vi "DC_CNTRL_step_HV.vi"(0 "Handle":u64, 1 "Ignore NACK":bool, 2 "Read Answer?":bool, 3 "Clear  RxTx Buffer?":bool, 5 "Box Number":u16(ring), 7 "Step (V)":dbl, 9 "Max Range (V)":dbl, 11 "error in (no error)":errorcluster) -> (4 "Handle out":u64, 15 "error out":errorcluster)   [LabVIEW 2019]
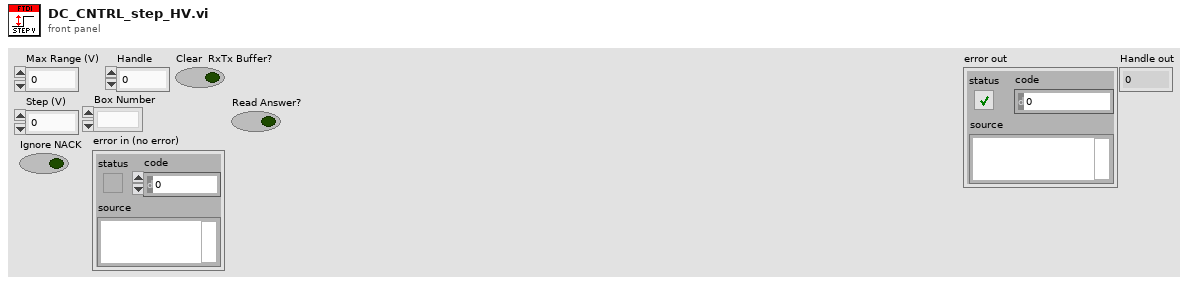
[diagram p1: front panel]
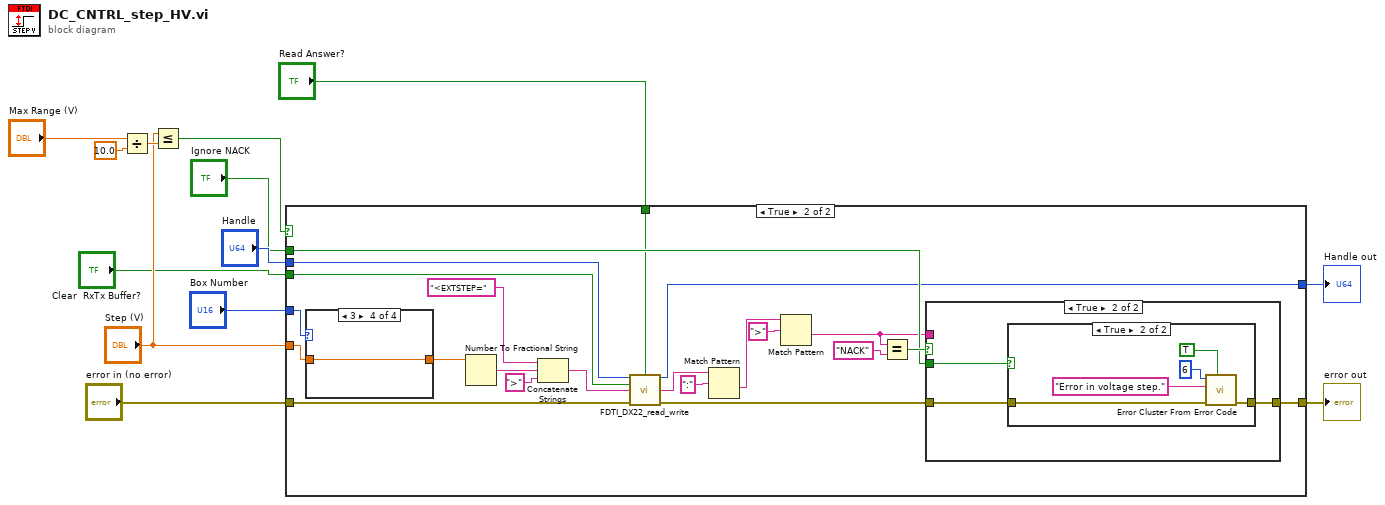
[diagram p0: block diagram]
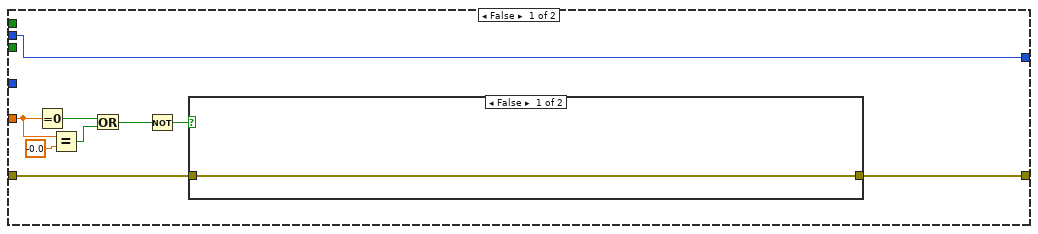
[diagram p2: hidden frame]
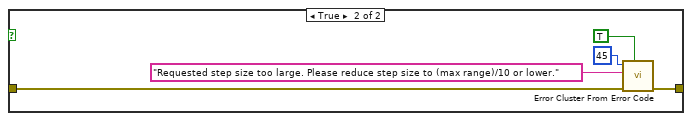
[diagram p3: hidden frame]
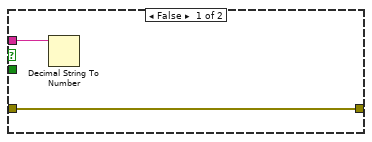
[diagram p4: hidden frame]
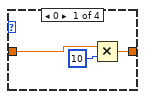
[diagram p6: hidden frame]
diagram:
  n1 = Divide(x="Max Range (V)", y=10.0) -> (x/y=w11:dbl)
  n2 = Less Or Equal?(x="Step (V)", y=w11) -> (x <= y?=w10:bool)
  n3 = case shown="True" w10 {
    tunnel: "Handle" -> [w14 w44]
    tunnel: "Box Number" -> [_ w50]
    tunnel: "Step (V)" -> [w21 w49]
    tunnel: "Ignore NACK" -> [_ w35]
    tunnel: [w17 w33] -> w3
    tunnel: "error in (no error)" -> [w18 w32]
    tunnel: "Clear  RxTx Buffer?" -> [_ w31]
    tunnel: [w14 w30] -> w2
    tunnel: "Read Answer?" -> [_ w29]
    frame False {
      n4 = Equal To 0?(x=w21) -> (x = 0?=w19:bool)
      n5 = Equal?(x=w21, y=-0.0) -> (x = y?=w20:bool)
      n6 = Or(x=w19, y=w20) -> (x .or. y?=w16:bool)
      n7 = Not(x=w16) -> (.not. x?=w15:bool)
      n8 = case shown="False" w15 {
        tunnel: w18 -> [w23 w28]
        tunnel: [w23 w24] -> w17
        frame False {
        }
        frame True {
          n9 = call <vilib>:"Error Cluster From Error Code.vi"("show call chain? (False)"=TRUE, "error in (no error)"=w28, "error message (\"\")"="Requested step size too large. Please reduce step size to (max range)/10 or lower." ("error message (\"\")"), "error code (0)"=45) -> ("error out"=w24:errorcluster)  [unwired: 5 in]
        }
      }
    }
    frame True {
      n10 = case shown="3" w50 {
        tunnel: w49 -> [w63 w65 w66 w67]
        tunnel: [w62 w65 w66 w67] -> w48
        frame 0 {
          n11 = Multiply(x=w63, y=u16 10) -> (x*y=w62:dbl)
        }
        frame 1, Default {
        }
        frame 2 {
        }
        frame 3 {
        }
      }
      n12 = Number To Fractional String(number=w48) -> (F-format string=w47:string)  [unwired: 3 in]
      n13 = Concatenate Strings("<EXTSTEP=" ("string"), w47, ">" ("string")) -> (w43:string)
      n14 = call "FDTI_DX22_read_write.vi"("Handle"=w44, "Read Answer?"=w29, "Clear  RxTx Buffer?"=w31, "Write string"=w43, "error in (no error)"=w32) -> ("Handle out"=w30:u64, "Read Data"=w42:string, "error out"=w36:errorcluster)  [unwired: 8 in]
      n15 = Match Pattern(string=w42, regular expression=":") -> (after substring=w40:string)  [unwired: 1 in, 3 out]
      n16 = Match Pattern(string=w40, regular expression=">") -> (after substring=w34:string)  [unwired: 1 in, 3 out]
      n17 = Equal?(x=w34, y="NACK") -> (x = y?=w37:bool)
      n18 = case shown="True" w37 {
        tunnel: w36 -> [w51 w54]
        tunnel: w35 -> [_ w55]
        tunnel: w34 -> [w52 _]
        tunnel: [w51 w53] -> w33
        frame False {
          n19 = Decimal String To Number(string=w52) -> ()  [unwired: 2 in, 2 out]
        }
        frame True {
          n20 = case shown="True" w55 {
            tunnel: w54 -> [w56 w61]
            tunnel: [w56 w58] -> w53
            frame False {
            }
            frame True {
              n21 = call <vilib>:"Error Cluster From Error Code.vi"("show call chain? (False)"=TRUE, "error in (no error)"=w61, "error message (\"\")"="Error in voltage step." ("error message (\"\")"), "error code (0)"=6) -> ("error out"=w58:errorcluster)  [unwired: 5 in]
            }
          }
        }
      }
    }
  }
  "error out" <- w3
  "Handle out" <- w2
